vi "Test3.vi"() -> ()   [LabVIEW 2017]
panel:
  in  "Boolean":bool
  in  "Numeric":dbl
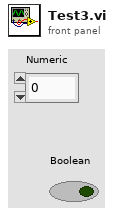
[diagram p1: front panel]
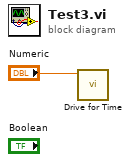
[diagram p0: block diagram]
diagram:
  n1 = call "Drive for Time.vi"("Left Speed"="Numeric") -> ()  [unwired: 9 in, 2 out]
